vi "Write One DAQ Waveform.vi"(7 "Offset in":u32, 8 "error in (no error)":errorcluster, 9 "Last Waveform":bool, 10 "Waveform Datatype":T1, 11 "CIPC Channel":u64) -> (0 "error out":errorcluster, 5 "Offset out":u32)   [LabVIEW 2021, in "CIF_CIPC_Fifo_DAQ.lvclass"]
uses:
  CIF_CIPC_Fifo_DAQ.lvclass
  ChannelCommon/typedef/Datatype Waveform.ctl
  ChannelCommon/typedef/Waveform Metadata.ctl
  <vilib>/CIF Foundation/CIF CIPC/TypeDefs/Partial Write Configuration.ctl
  296b4b7f-f24e-461b-ac09-61c48c94f223.vi
  489ce88f-d13b-4e3d-8a44-beac6fbb575f.vi
  <vilib>/CIF Foundation/CIF CIPC/SubVIs/Check Error.vi
  <vilib>/CIF Foundation/CIF CIPC/SubVIs/Notify Of New Write.vi
  <vilib>/CIF Foundation/CIF CIPC/SubVIs/Get dll Path.vi
  <vilib>/CIF Foundation/CIF CIPC/SubVIs/Get Element Write Position.vi
  <vilib>/Utility/error.llb/Trim Whitespace.vi
  <vilib>/Utility/error.llb/Error Cluster From Error Code.vi
  CIF_CIPC_Fifo_DAQ.lvclass/CIF_CIPC_Fifo_DAQ.ctl
  <vilib>/CIF Foundation/CIF CIPC/CIF_NI_CIPC.lvlib
  ChannelCommon/ChannelCommon.lvlib
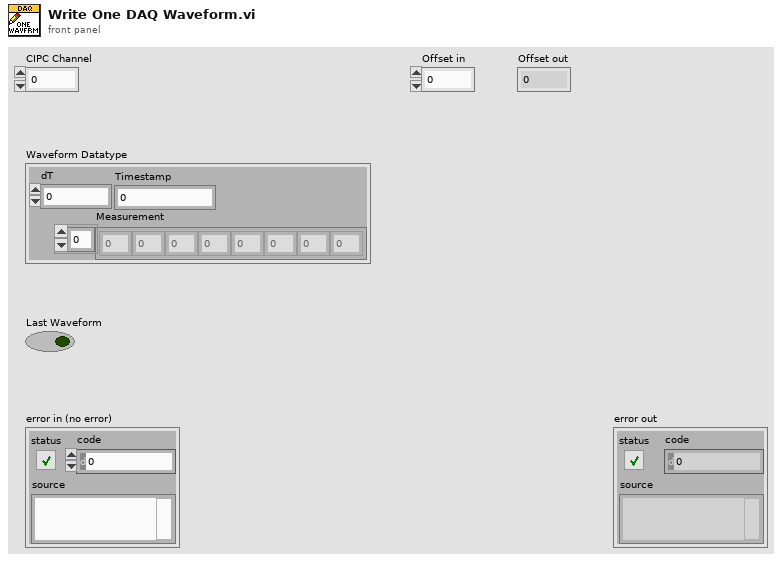
[diagram p1: front panel]
types:
  T1 = typedef "ChannelCommon.lvlib/Datatype Waveform.ctl" = cluster{"Measurement":dbl[], "dT":dbl, "Timestamp":i64}
  T2 = typedef "ChannelCommon.lvlib/Waveform Metadata.ctl" = cluster{"Timestamp":i64, "dT":dbl, "Array Length":u64}
  T3 = typedef "CIF_NI_CIPC.lvlib/Partial Write Configuration.ctl" = cluster{"Start Offset (bytes)":u32, "Total Length (bytes)":u32, "Last Write":bool, "Get Write Position":bool, "Notify Readers":bool}
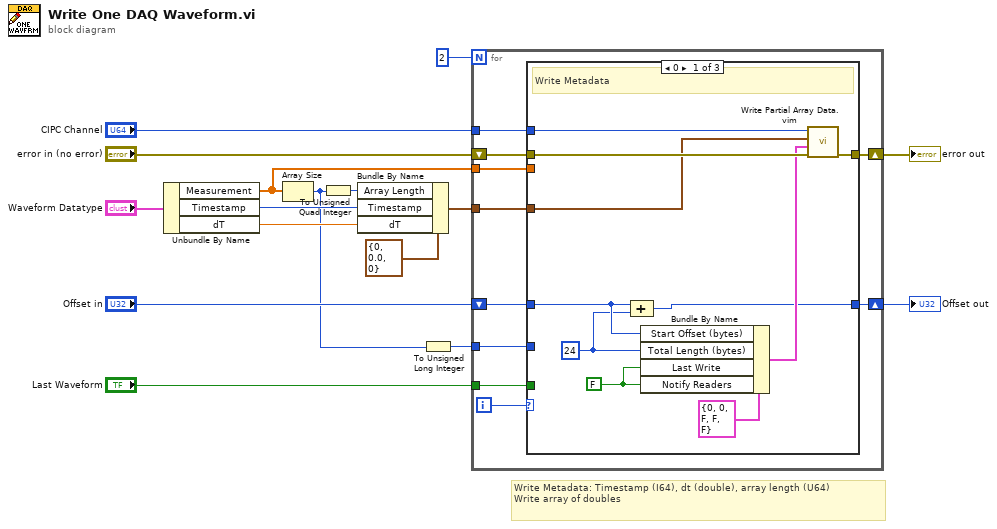
[diagram p0: block diagram]
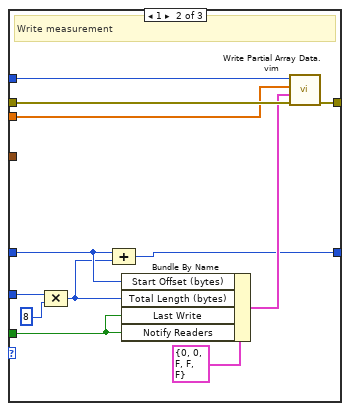
[diagram p2: hidden frame]
diagram:
  # "Write Metadata: Timestamp (I64), dt (double), array length (U64)\nWrite array of doubles"
  n1 = Unbundle By Name("Waveform Datatype") -> ("Measurement"=w3:dbl[], "Timestamp"=w7:i64, "dT"=w6:dbl)
  n2 = Array Size(array=w3) -> (size(s)=w1:i32)
  n3 = To Unsigned Quad Integer(1:w1) -> (0:w4:u64)
  n4 = Bundle By Name(cluster=T2 {"Timestamp"=0, "dT"=0.0, "Array Length"=0} ("Waveform Meta Data"), "Array Length"=w4, "Timestamp"=w7, "dT"=w6) -> (w5:T2)
  n5 = To Unsigned Long Integer(number=w1) -> (unsigned 32bit integer=w2:u32)
  n6 = for {
    N: 2 -> [_]
    tunnel: "CIPC Channel" -> [w26]
    shift-right: [w24] -> w11
    shift-left: "error in (no error)" -> [w25]
    shift-right: [w21] -> w13
    shift-left: "Offset in" -> [w23]
    tunnel: "Last Waveform" -> [w20]
    tunnel: w2 -> [w19]
    tunnel: w5 -> [w18]
    tunnel: w3 -> [w17]
    i -> [w22]
    n7 = case shown="0" w22 {
      tunnel: w26 -> [w36 w48 _]
      tunnel: w25 -> [w35 w47 w50]
      tunnel: [w34 w46 w50] -> w24
      tunnel: w23 -> [w31 w43 w49]
      tunnel: [w30 w42 w49] -> w21
      tunnel: w20 -> [_ w41 _]
      tunnel: w19 -> [_ w40 _]
      tunnel: w18 -> [w27 _ _]
      tunnel: w17 -> [_ w37 _]
      frame 0 {
        w28 = FALSE ("Last Write")
        w29 = u32 24 ("Total Length (bytes)")
        # "Write Metadata"
        n8 = Compound Arithmetic op=ADD(w31, w29) -> (w30:u32)
        n9 = Bundle By Name(cluster=T3 {"Start Offset (bytes)"=0, "Total Length (bytes)"=0, "Last Write"=FALSE, "Get Write Position"=FALSE, "Notify Readers"=FALSE} ("Partial Write Configuration"), "Start Offset (bytes)"=w31, "Total Length (bytes)"=w29, "Last Write"=w28, "Notify Readers"=w28) -> (w32:T3)
        n10 = call "Write Partial Array Data.vim"("error in (no error)"=w35, "Partial Write Configuration"=w32, "Data in"=w27, "CIPC Reference in"=w36) -> ("error out"=w34:errorcluster)  [unwired: 4 in, 3 out]
      }
      frame 1 {
        # "Write measurement"
        n11 = Compound Arithmetic op=MULTIPLY(w40, u32 8 ("Total Length (bytes)")) -> (w38:u32)
        n12 = Compound Arithmetic op=ADD(w43, w38) -> (w42:u32)
        n13 = Bundle By Name(cluster=T3 {"Start Offset (bytes)"=0, "Total Length (bytes)"=0, "Last Write"=FALSE, "Get Write Position"=FALSE, "Notify Readers"=FALSE} ("Partial Write Configuration"), "Start Offset (bytes)"=w43, "Total Length (bytes)"=w38, "Last Write"=w41, "Notify Readers"=w41) -> (w44:T3)
        n14 = call "Write Partial Array Data.vim"("error in (no error)"=w47, "Partial Write Configuration"=w44, "Data in"=w37, "CIPC Reference in"=w48) -> ("error out"=w46:errorcluster)  [unwired: 4 in, 3 out]
      }
      frame 2, Default {
        # "Default"
      }
    }
  }
  "Offset out" <- w13
  "error out" <- w11
